vi "Helium Configuration to Strings.vi"(11 "Test Information":T1) -> (2 "Thresholds":string[][](array[string]), 3 "Timings":string[][](array[string]))   [LabVIEW 2015]
uses:
  Tests/Controls/Test Information.ctl
  Tests/Controls/Vacuum Test.ctl
  Tests/Controls/Test Timing.ctl
  Tests/Controls/Vaccum Thresholds.ctl
  Tests/Controls/Helium Test.ctl
  Tests/Controls/Helium Thresholds.ctl
  Tests/Controls/Startup Thresholds.ctl
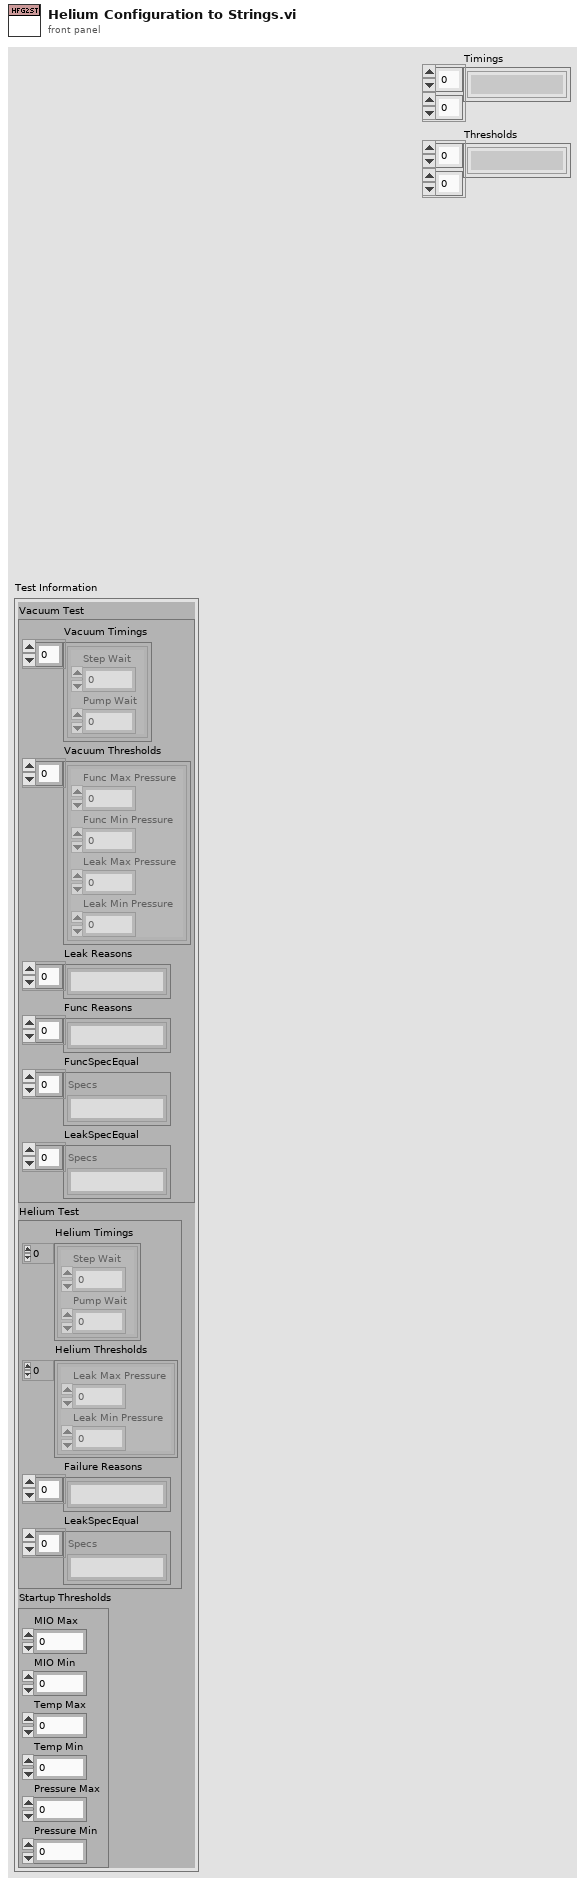
[diagram p1: front panel]
types:
  T1 = typedef "Test Information.ctl" = cluster{"Vacuum Test":T2, "Helium Test":T5, "Startup Thresholds":T7}
  T2 = typedef "Vacuum Test.ctl" = cluster{"Vacuum Timings":T3[], "Vacuum Thresholds":T4[], "Leak Reasons":string[], "Func Reasons":string[], "FuncSpecEqual":string[], "LeakSpecEqual":string[]}
  T3 = typedef "Test Timing.ctl" = cluster{"Step Wait":dbl, "Pump Wait":dbl}
  T4 = typedef "Vaccum Thresholds.ctl" = cluster{"Func Max Pressure":dbl, "Func Min Pressure":dbl, "Leak Max Pressure":dbl, "Leak Min Pressure":dbl}
  T5 = typedef "Helium Test.ctl" = cluster{"Helium Timings":T3[], "Helium Thresholds":T6[], "Failure Reasons":string[], "LeakSpecEqual":string[]}
  T6 = typedef "Helium Thresholds.ctl" = cluster{"Leak Max Pressure":dbl, "Leak Min Pressure":dbl}
  T7 = typedef "Startup Thresholds.ctl" = cluster{"MIO Max":dbl, "MIO Min":dbl, "Temp Max":dbl, "Temp Min":dbl, "Pressure Max":dbl, "Pressure Min":dbl}
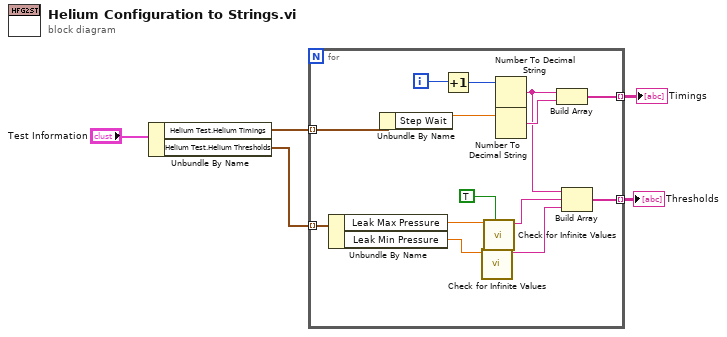
[diagram p0: block diagram]
diagram:
  n1 = Unbundle By Name("Test Information") -> ("Helium Test.Helium Timings"=w5:T3[], "Helium Test.Helium Thresholds"=w3:T6[])
  n2 = for {
    tunnel: w5 -> [w19] mode=indexing
    tunnel: [w16] -> w4 mode=indexing
    tunnel: w3 -> [w13] mode=indexing
    tunnel: [w11] -> w2 mode=indexing
    i -> [w18]
    n3 = Unbundle By Name(w13) -> ("Leak Max Pressure"=w10:dbl, "Leak Min Pressure"=w7:dbl)
    n4 = Unbundle By Name(w19) -> ("Step Wait"=w15:dbl)
    n5 = Increment(x=w18) -> (x+1=w17:i32)
    n6 = call "Check for Infinite Values.vi"("Pressure Limit"=w7) -> ("element"=w6:string)  [unwired: 10 in]
    n7 = call "Check for Infinite Values.vi"("Positive?"=TRUE, "Pressure Limit"=w10) -> ("element"=w8:string)  [unwired: 9 in]
    n8 = Number To Decimal String(number=w17) -> (decimal integer string=w12:string)  [unwired: 1 in]
    n9 = Number To Decimal String(number=w15) -> (decimal integer string=w14:string)  [unwired: 1 in]
    n10 = Build Array(w12, w14) -> (w16:string[])
    n11 = Build Array(w12, w8, w6) -> (w11:string[])
  }
  "Timings" <- w4
  "Thresholds" <- w2
